vi "From String Array.vi"(8 "error in (no error)":errorcluster, 9 "String Array":string[](array[string]), 11 "Numeric Limit Compare Config in":refnum<class "Numeric Limit Compare Config.lvclass">) -> (0 "error out":errorcluster, 1 "String Array 2":string[](array[string]), 2 "Version":string, 3 "Numeric Limit Compare Config out":refnum<class "Numeric Limit Compare Config.lvclass">)   [LabVIEW 2015, in "Numeric Limit Compare Config.lvclass"]
uses:
  Numeric Limit Compare Config.lvclass
  <vilib>/NI/Tag Bus/tag/Data Type.ctl
  <vilib>/NI/Tag Bus Module Framework/channel/channel classification.ctl
  Comparison Types.ctl
  Numeric Limit Compare Config.lvclass/Numeric Limit Compare Config.ctl
  Write channel.vi
  Write Result Channel.vi
  Write Comparison Type.vi
  Write Negate Result.vi
  Write Upper Limit_Limit.vi
  Write Lower Limit.vi
  classes/Step/Config/Step Config.lvclass
  <vilib>/NI/Tag Bus Module Framework/channel/TBM channel.lvclass
  <vilib>/NI/Tag Bus/tag/tag descriptor.lvclass
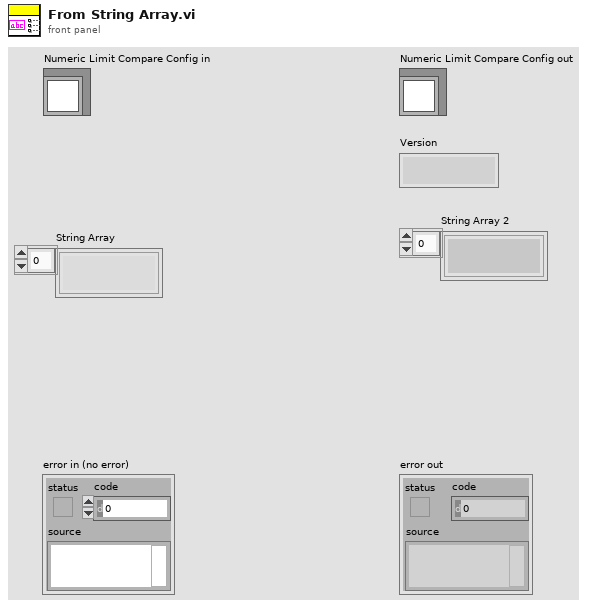
[diagram p1: front panel]
types:
  T1 = typedef "TBM channel.lvclass/channel classification.ctl" = enum16{"input data", "output data", "processing parameter", "processing result"}
  T2 = typedef "tag bus.lvlib/tag descriptor.lvclass/Data Type.ctl" = enum16{"Double", "Single", "I64", "I32", "I16", "I8", "U64", "U32", "U16", "U8", "Boolean", "String", "Array of Double", "Array of Single", "Array of I64", "Array of I32", "Array of I16", "Array of I8", "Array of U64", "Array of U32", "Array of U16", "Array of U8", "Array of Boolean", "Array of String"}
  T3 = typedef "Comparison Types.ctl" = enum16{"GELE (>=<=)", "GTLE(><=)", "GTLT(><)", "GELT(>=<)", "EQ(==)", "NE (!=)", "GT(>)", "LT(<)", "GE(>=)", "LE(<=)"}
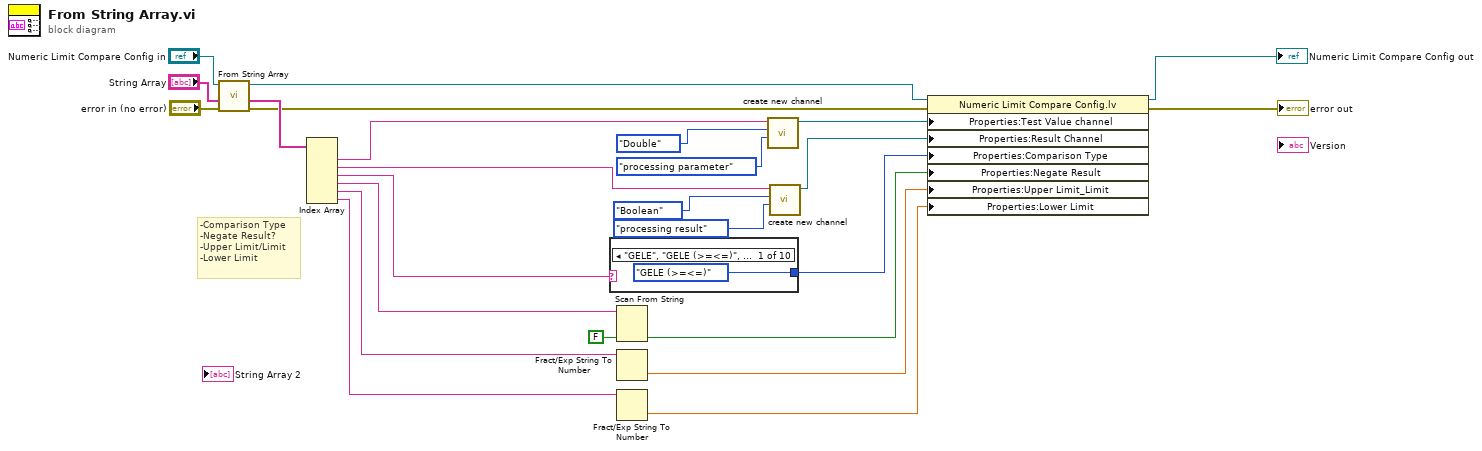
[diagram p0: block diagram]
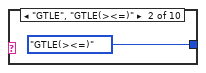
[diagram p2: hidden frame]
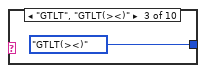
[diagram p3: hidden frame]
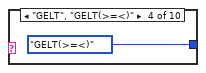
[diagram p4: hidden frame]
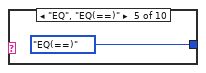
[diagram p5: hidden frame]
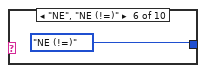
[diagram p6: hidden frame]
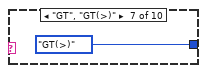
[diagram p7: hidden frame]
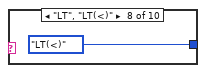
[diagram p8: hidden frame]
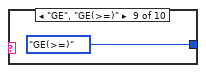
[diagram p9: hidden frame]
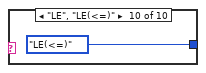
[diagram p10: hidden frame]
diagram:
  # "-Comparison Type\n-Negate Result?\n-Upper Limit/Limit\n-Lower Limit"
  n1 = call-parent "From String Array.vi"("error in (no error)"="error in (no error)", "String Array"="String Array", "Step Config in"="Numeric Limit Compare Config in") -> ("error out"=w17:errorcluster, "Elements Left"=w22:string[], "Step Config out"=w19:refnum<class "Numeric Limit Compare Config.lvclass">)  [unwired: 5 in, 1 out]
  n2 = Index Array(array=w22) -> (element #1=w2:string, element #2=w1:string, element #3=w3:string, element #4=w4:string, element #5=w5:string, element #6=w6:string)  [unwired: 6 in]
  n3 = case shown="\"GELE\", \"GELE (>=<=)\", Default" w3 {
    tunnel: [Comparison_Types."GELE (>=<=)" ("Comparison Type") Comparison_Types."GTLE(><=)" ("Comparison Type") Comparison_Types."GTLT(><)" ("Comparison Type") Comparison_Types."GELT(>=<)" ("Comparison Type") Comparison_Types."EQ(==)" ("Comparison Type") Comparison_Types."NE (!=)" ("Comparison Type") Comparison_Types."GT(>)" ("Comparison Type") Comparison_Types."LT(<)" ("Comparison Type") Comparison_Types."GE(>=)" ("Comparison Type") Comparison_Types."LE(<=)" ("Comparison Type")] -> w16
    frame "GELE", "GELE (>=<=)", Default {
    }
    frame "GTLE", "GTLE(><=)" {
    }
    frame "GTLT", "GTLT(><)" {
    }
    frame "GELT", "GELT(>=<)" {
    }
    frame "EQ", "EQ(==)" {
    }
    frame "NE", "NE (!=)" {
    }
    frame "GT", "GT(>)" {
    }
    frame "LT", "LT(<)" {
    }
    frame "GE", "GE(>=)" {
    }
    frame "LE", "LE(<=)" {
    }
  }
  n4 = Scan From String(input string=w4, default 1=FALSE ("Negate Result")) -> (output 1=w15:bool)  [unwired: 3 in, 3 out]
  n5 = Fract/Exp String To Number(string=w5) -> (number=w13:dbl)  [unwired: 3 in, 1 out]
  n6 = Fract/Exp String To Number(string=w6) -> (number=w12:dbl)  [unwired: 3 in, 1 out]
  n7 = call <vilib>:"create new channel.vi"("channel classification"=channel_classification."processing parameter", "data type"=Data_Type."Double", "channel name"=w2) -> ("channel"=w18:refnum<class "TBM channel.lvclass">)  [unwired: 8 in]
  n8 = call <vilib>:"create new channel.vi"("channel classification"=channel_classification."processing result", "data type"=Data_Type."Boolean", "channel name"=w1) -> ("channel"=w7:refnum<class "TBM channel.lvclass">)  [unwired: 8 in]
  n9 = property class="Numeric Limit Compare Config.lv"(reference=w19, error in=w17, "Properties:Test Value channel"=w18, "Properties:Result Channel"=w7, "Properties:Comparison Type"=w16, "Properties:Negate Result"=w15, "Properties:Upper Limit_Limit"=w13, "Properties:Lower Limit"=w12) -> (reference out=→"Numeric Limit Compare Config out":refnum<class "Numeric Limit Compare Config.lvclass">, error out=→"error out":errorcluster)
